vi "Project Items - Get Owned Items.vi"(8 "Error In":errorcluster, 11 "Project Item":refnum<vi>) -> (0 "Error Out":errorcluster, 3 "Owned Items":refnum<vi>[](array[refnum]))   [LabVIEW 2022 SP3]
doc: "<add documentation here>"
panel:
  # "Development\nControls or indicators that are useful for development or testing, but which are not outputs of the VI."
  # "Input\nInputs to the VI"
  # "Output\nOutputs of the VI"
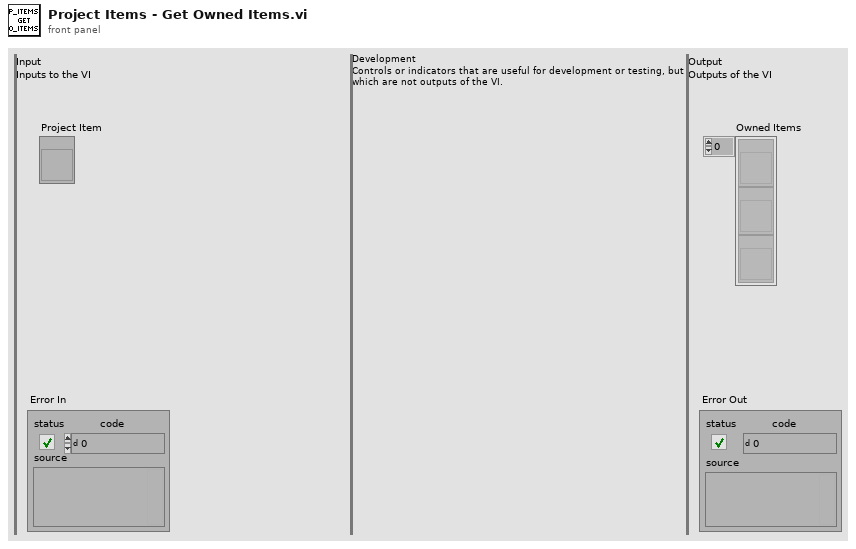
[diagram p1: front panel]
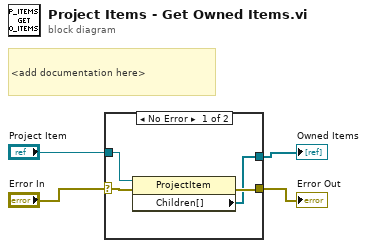
[diagram p0: block diagram]
diagram:
  # "<add documentation here>"
  n1 = case shown="No Error" "Error In" {
    selector: "Error In" -> [w8 w9]
    tunnel: [w6 w9] -> w3
    tunnel: "Project Item" -> [w7 _]
    tunnel: [w5 _] -> w1
    frame No Error {
      n2 = property class="ProjectItem"(reference=w7, error in=w8) -> (error out=w6:errorcluster, "Children[]"=w5:refnum<vi>[])  [unwired: 1 out]
    }
    frame Error {
    }
  }
  "Error Out" <- w3
  "Owned Items" <- w1
